vi "#86-2017.vi"() -> ()   [LabVIEW 2017]
uses:
  6f3e7e63-859a-43a6-8964-4616b90ac9e5.vi
  ee8334f3-fe61-4e76-b193-819b6ef244fc.vi
  API-String-Arugments-Support/_Support/Data To API String Arguments.vi
  API-String-Arugments-Support/_Support/Convert API String Arguments to Data(variant).vi
panel:
  in  "Cluster":T1={"1"=TRUE, "2"=[2, 2], "3"={"3.1"="3.1", "3.2"=3.2, "3.3"=TRUE}, "5"={"5.2"=TRUE}}
  out "String":string
  out "Data":T2
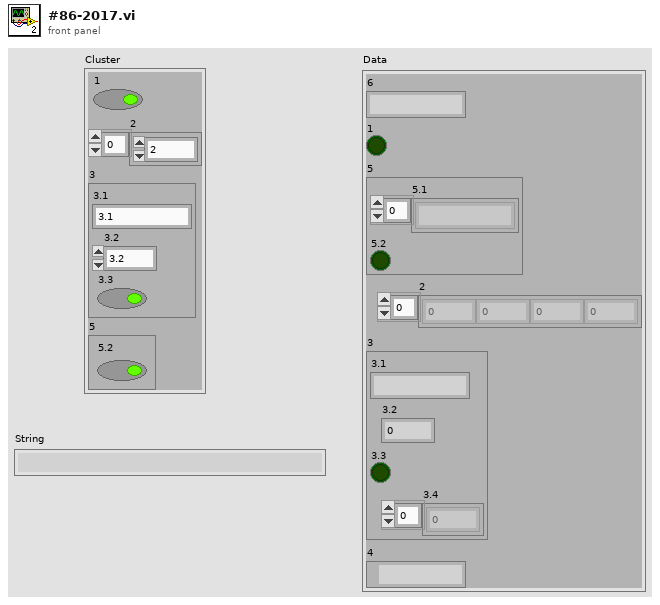
[diagram p1: front panel]
types:
  T1 = cluster{"1":bool, "2":i32[], "3":cluster{"3.1":string, "3.2":dbl, "3.3":bool}, "5":cluster{"5.2":bool}}
  T2 = cluster{"6":string, "1":bool, "5":cluster{"5.1":string[], "5.2":bool}, "2":i32[], "3":cluster{"3.1":string, "3.2":dbl, "3.3":bool, "3.4":i32[]}, "4":path}
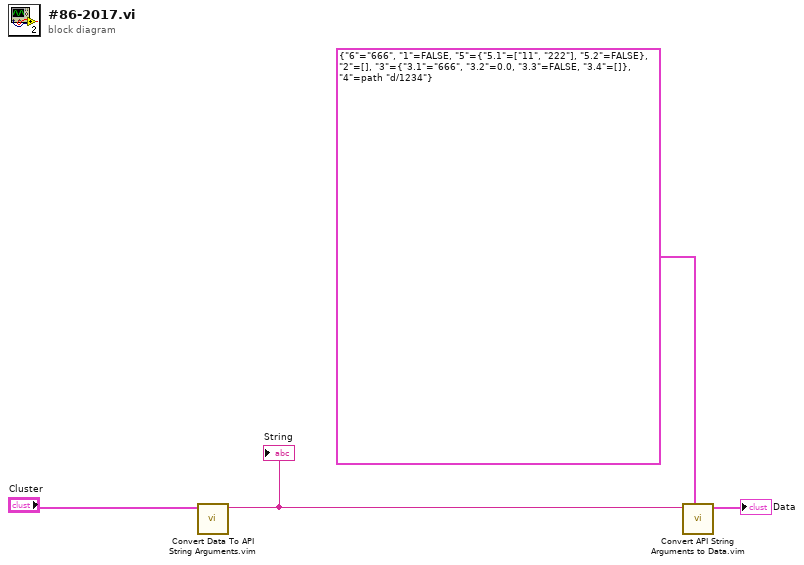
[diagram p0: block diagram]
diagram:
  n1 = call "Convert Data To API String Arguments.vim"("data"="Cluster") -> ("String"=w3:string)  [unwired: 7 in, 1 out]
  "String" <- w3
  n2 = call "Convert API String Arguments to Data.vim"("Type"=T2 {"6"="666", "1"=FALSE, "5"={"5.1"=["11", "222"], "5.2"=FALSE}, "2"=[], "3"={"3.1"="666", "3.2"=0.0, "3.3"=FALSE, "3.4"=[]}, "4"=path "d:/1234"}, "String"=w3) -> ("Data"=→"Data":T2)  [unwired: 6 in, 1 out]
